vi "Climber_Hardware_Begin.vi"   [LabVIEW 2020]
uses:
  Climber_Hardware_Globals.vi
  <vilib>/Rock Robotics/WPI/ThirdParty/Phoenix-LabVIEW/Motor Controller/Controls/CTRE_Phoenix_MotorControl_TalonFXInvertType.ctl
types:
  T1 = typedef "CTRE_Phoenix_MotorControl_TalonFXInvertType.ctl" = enum16{"Counter-Clockwise", "Clockwise"}
  T2 = typedef "WPI_MotorControlDeviceRef.ctl" = cluster{"DeviceStatus":errorcluster, "Type":T3, "PWM":cluster{"PWM Channel":T4, "DeadBand":T5}, "CAN":cluster{"Device Number":u8, "SetOutput VI Ref":variant, "GetOutput VI Ref":variant, "Enable VI Ref":variant, "Disable VI Ref":variant, "Data":variant}, "Invert":bool, "DIO PWM":cluster{"PWM \"Enable\" Channel":T4, "DIOChannel":T6, "PWM Rate":dbl}}
  T3 = typedef "WPI_MotorControlType.ctl" = enum16{"PWM", "CAN", "DIO PWM"}
  T4 = typedef "FPGA_DIOPWMChannel.ctl" = enum8{"PWM 0", "PWM 1", "PWM 2", "PWM 3", "PWM 4", "PWM 5", "PWM 6", "PWM 7", "PWM 8", "PWM 9", "PWM MXP 0", "PWM MXP 1", "PWM MXP 2", "PWM MXP 3", "PWM MXP 4", "PWM MXP 5", "PWM MXP 6", "PWM MXP 7", "PWM MXP 8", "PWM MXP 9", "Invalid"}
  T5 = typedef "WPI_PWMDeadband.ctl" = cluster{"Name":string, "maxPositivePwm":i32, "minPositivePwm":i32, "centerPwm":i32, "maxNegativePwm":i32, "minNegativePwm":i32, "angularRange":u16}
  T6 = typedef "FPGA_DIOChannel.ctl" = enum8{"DIO 0", "DIO 1", "DIO 2", "DIO 3", "DIO 4", "DIO 5", "DIO 6", "DIO 7", "DIO 8", "DIO 9", "DIO MXP 0", "DIO MXP 1", "DIO MXP 2", "DIO MXP 3", "DIO MXP 4", "DIO MXP 5", "DIO MXP 6", "DIO MXP 7", "DIO MXP 8", "DIO MXP 9", "DIO MXP 10", "DIO MXP 11", "DIO MXP 12", "DIO MXP 13", "DIO MXP 14", "DIO MXP 15", "SPI Port CS1", "SPI Port CS2", "SPI Port CS3", "SPI Port MISO", "SPI Port MOSI", "Invalid"}
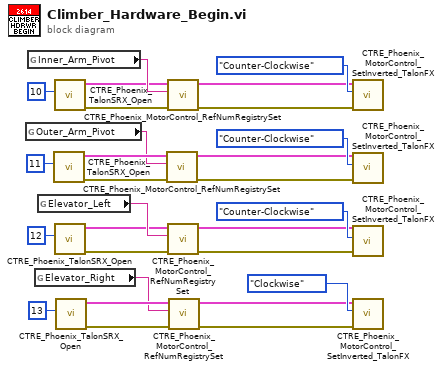
[diagram p0: block diagram]
diagram:
  n1 = global read "Climber_Hardware_Globals.vi" "Outer_Arm_Pivot"() -> (w5:string)
  n2 = global read "Climber_Hardware_Globals.vi" "Inner_Arm_Pivot"() -> (w4:string)
  n3 = global read "Climber_Hardware_Globals.vi" "Elevator_Right"() -> (w13:string)
  n4 = global read "Climber_Hardware_Globals.vi" "Elevator_Left"() -> (w12:string)
  n5 = call <vilib>:"CTRE_Phoenix_TalonSRX_Open.vi"("Device Number"=u8 11) -> ("error out"=w7:errorcluster, "PhoenixMotorControlDevRef"=w6:T2)  [unwired: 9 in]
  n6 = call <vilib>:"CTRE_Phoenix_TalonSRX_Open.vi"("Device Number"=u8 10) -> ("error out"=w2:errorcluster, "PhoenixMotorControlDevRef"=w3:T2)  [unwired: 9 in]
  n7 = call <vilib>:"CTRE_Phoenix_TalonSRX_Open.vi"("Device Number"=u8 12) -> ("error out"=w10:errorcluster, "PhoenixMotorControlDevRef"=w11:T2)  [unwired: 9 in]
  n8 = call <vilib>:"CTRE_Phoenix_TalonSRX_Open.vi"("Device Number"=u8 13) -> ("error out"=w15:errorcluster, "PhoenixMotorControlDevRef"=w14:T2)  [unwired: 9 in]
  n9 = call <vilib>:"CTRE_Phoenix_MotorControl_RefNumRegistrySet.vi"("error in (no error)"=w7, "refnum name"=w5, "PhoenixMotorControlDevRef"=w6) -> ("error out"=w20:errorcluster, "PhoenixMotorControlDevRef"=w19:T2)  [unwired: 7 in]
  n10 = call <vilib>:"CTRE_Phoenix_MotorControl_RefNumRegistrySet.vi"("error in (no error)"=w2, "refnum name"=w4, "PhoenixMotorControlDevRef"=w3) -> ("error out"=w17:errorcluster, "PhoenixMotorControlDevRef"=w18:T2)  [unwired: 7 in]
  n11 = call <vilib>:"CTRE_Phoenix_MotorControl_RefNumRegistrySet.vi"("error in (no error)"=w10, "refnum name"=w12, "PhoenixMotorControlDevRef"=w11) -> ("error out"=w22:errorcluster, "PhoenixMotorControlDevRef"=w21:T2)  [unwired: 7 in]
  n12 = call <vilib>:"CTRE_Phoenix_MotorControl_RefNumRegistrySet.vi"("error in (no error)"=w15, "refnum name"=w13, "PhoenixMotorControlDevRef"=w14) -> ("error out"=w24:errorcluster, "PhoenixMotorControlDevRef"=w23:T2)  [unwired: 7 in]
  n13 = call <vilib>:"CTRE_Phoenix_MotorControl_SetInverted_TalonFX.vi"("error in (no error)"=w17, "Invert Type"=CTRE_Phoenix_MotorControl_TalonFXInvertType."Counter-Clockwise", "PhoenixMotorControlDevRef"=w18) -> ()  [unwired: 7 in, 2 out]
  n14 = call <vilib>:"CTRE_Phoenix_MotorControl_SetInverted_TalonFX.vi"("error in (no error)"=w20, "Invert Type"=CTRE_Phoenix_MotorControl_TalonFXInvertType."Counter-Clockwise", "PhoenixMotorControlDevRef"=w19) -> ()  [unwired: 7 in, 2 out]
  n15 = call <vilib>:"CTRE_Phoenix_MotorControl_SetInverted_TalonFX.vi"("error in (no error)"=w22, "Invert Type"=CTRE_Phoenix_MotorControl_TalonFXInvertType."Counter-Clockwise", "PhoenixMotorControlDevRef"=w21) -> ()  [unwired: 7 in, 2 out]
  n16 = call <vilib>:"CTRE_Phoenix_MotorControl_SetInverted_TalonFX.vi"("error in (no error)"=w24, "Invert Type"=CTRE_Phoenix_MotorControl_TalonFXInvertType."Clockwise", "PhoenixMotorControlDevRef"=w23) -> ()  [unwired: 7 in, 2 out]
